vi "Parse Response (Object).vi"(8 "error in":errorcluster, 10 "Response String In":string) -> (0 "error out":errorcluster, 1 "LabVIEW Error?":bool=TRUE, 2 "JSON Array":refnum<class "JSON Object.lvclass">)   [LabVIEW 2016, in "JSONRPC Server.lvclass"]
uses:
  JSONRPC Server.lvclass
  <vilib>/NI/JSON Support for LabVIEW/JSON Data Classes/JSON Object/JSON Object.lvclass
  <vilib>/NI/JSON Support for LabVIEW/JSON Data Classes/JSON Helper/To More Specific Type (Object).vi
  <vilib>/NI/JSON Support for LabVIEW/JSON Data Classes/JSON Helper/JSON Helper.lvclass
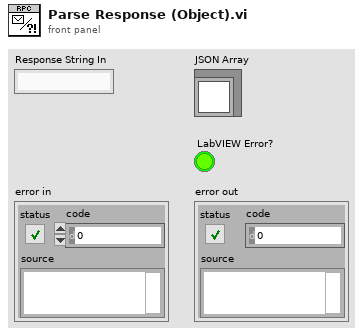
[diagram p1: front panel]
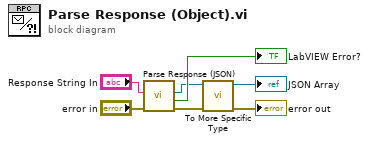
[diagram p0: block diagram]
diagram:
  n1 = call "Parse Response (JSON).vi"("error in"="error in", "Response String In"="Response String In") -> ("error out"=w3:errorcluster, "LabVIEW Error?"=→"LabVIEW Error?":bool, "JSON out"=w4:refnum<class "JSON Null.lvclass">)  [unwired: 7 in]
  n2 = call-poly <vilib>:"To More Specific Type.vi"("error in (no error)"=w3, "JSON Datatype in"=w4) -> ("error out"=→"error out":errorcluster, "JSON Datatype out"=→"JSON Array":refnum<class "JSON Object.lvclass">)  [unwired: 8 in]
